vi "Run_2_of_6_Tests.vi"() -> ()   [LabVIEW 2019]
uses:
  <vilib>/Rock Robotics/WPI/ThirdParty/JAS_Junk/TrajLib/Trajectory_Library.lvlib
panel:
  out "Meca Drive \nOdometry":bool
  out "Meca Drive \nKinematics":bool
  out "String":string
  out "Flywheel Simulation":bool
  out "Matrix":bool
  out "PID":bool
  out "Math Utils":bool
  out "Linear Filter":bool
  out "Linear System Loop":bool
  out "All Tests Finished":bool
  out "Holonomic Drive Ctrl":bool
  out "Linear Plant Inv FF":bool
  out "Numerical Jacobian":bool
  out "Merwe Scaled Sigma Pts":bool
  out "Numerical Integration":bool
  out "Median Filter":bool
  out "Linear System ID":bool
  out "Kalman filter":bool
  out "PID Input / Output":bool
  out "Linear Quadradtic Regulator":bool
  # "FORMAL TRAJECTORY / CONTROL LIBRARY TEST PROCEDURE"
  # "FUNCTION NOT\nIMPLEMENTED"
  # "Extended Kalman Filter"
  # "FUNCTION NOT\nIMPLEMENTED"
  # "Meca Drive Pose Est"
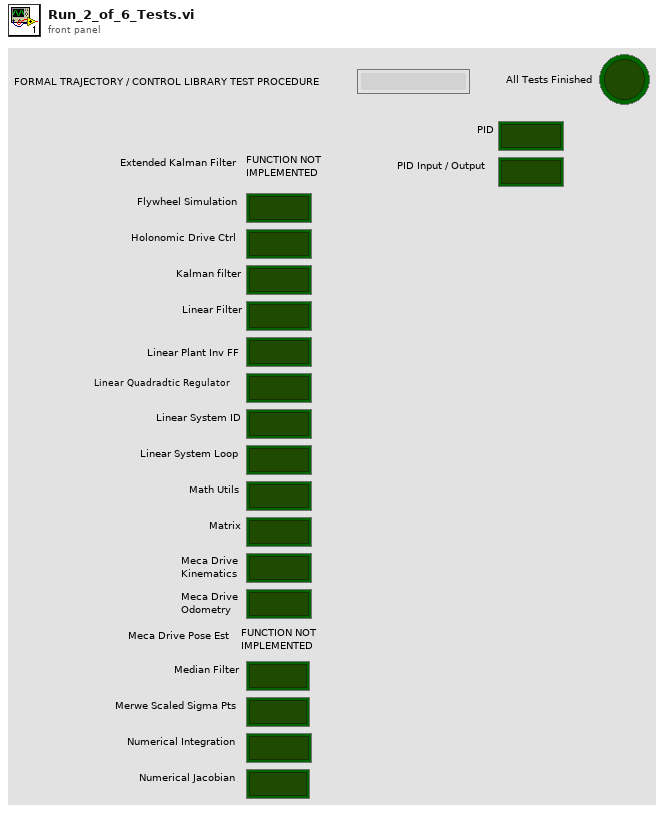
[diagram p1: front panel]
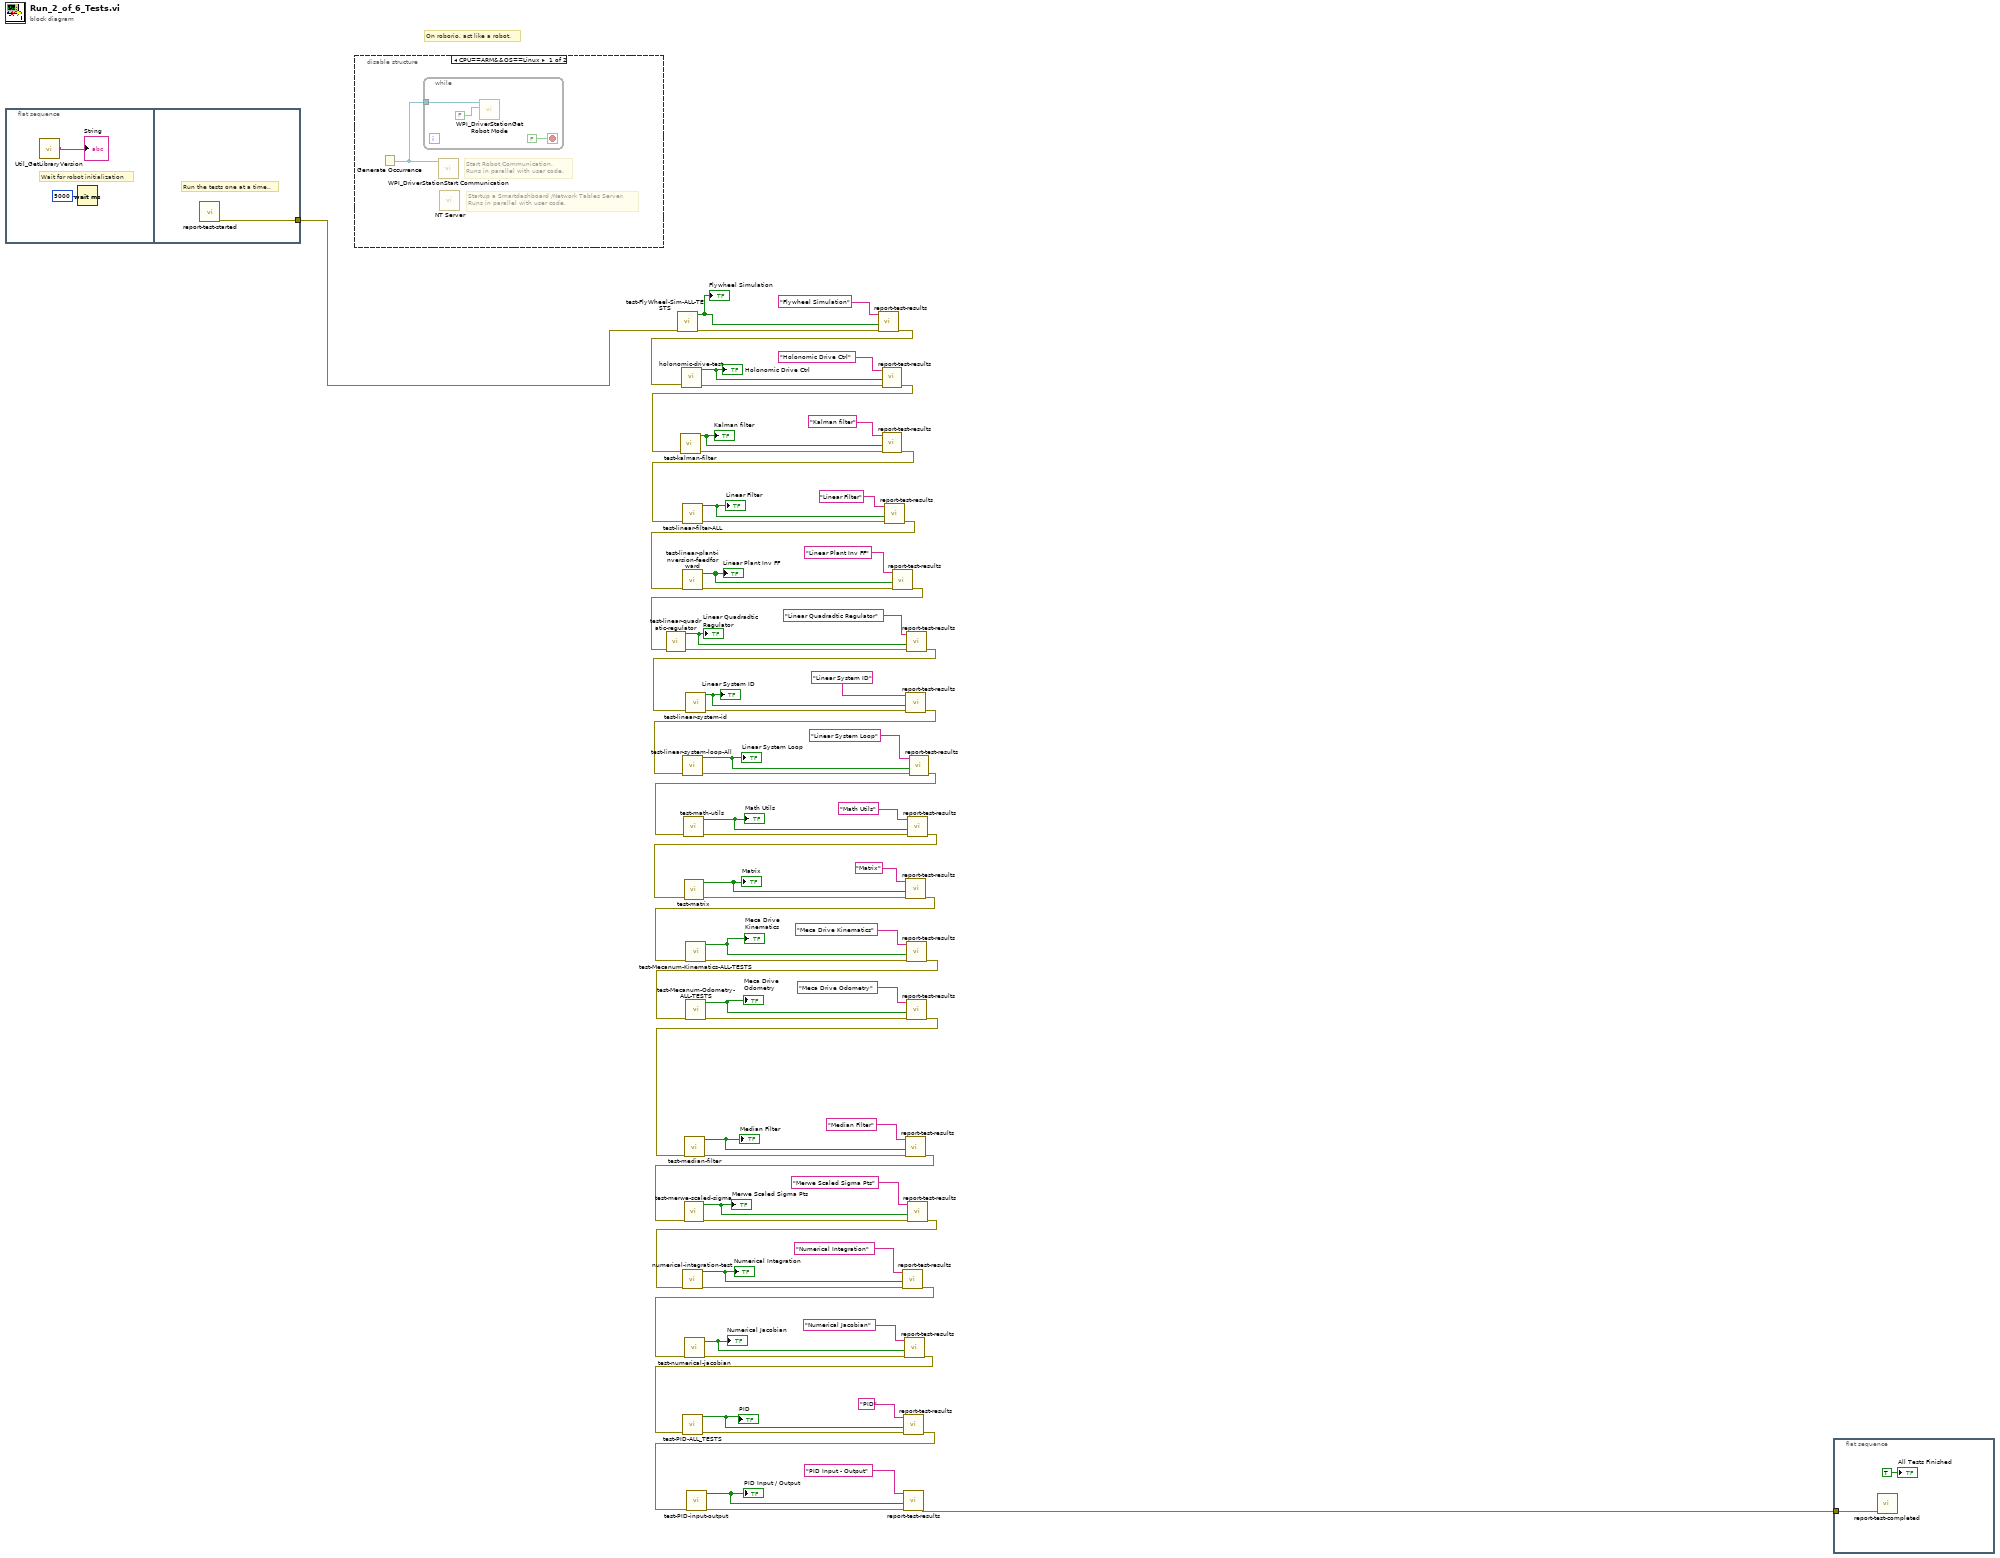
[diagram p0: block diagram]
diagram:
  # "On roborio, act like a robot."
  n1 = flat-sequence {
    tunnel: [w76] -> w12
    frame #0 {
      # "Wait for robot initialization"
      n2 = call <vilib>:"Util_GetLibraryVersion.vi"() -> ("TrajLibVersion"=→"String":string)  [unwired: 11 in]
      n3 = Wait (ms)(milliseconds to wait=u32 5000) -> ()  [unwired: 1 out]
    }
    frame #1 {
      # "Run the tests one at a time.."
      n4 = call "report-test-started.vi"() -> ("error out"=w76:errorcluster)  [unwired: 11 in]
    }
  }
  n5 = disable-structure shown="CPU==ARM&&OS==Linux" {
    frame condition #0 {
      # "Startup a Smartdashboard /Network Tables Server.\nRuns in parallel with user code."
      # "Start Robot Communication.\nRuns in parallel with user code."
      n6 = Generate Occurrence() -> (w77:refnum<k4>)
      n7 = while {
        tunnel: w77 -> [w80]
        stop <- FALSE stop-if-true
        n8 = call <vilib>:"WPI_DriverStationGet Robot Mode.vi"("Finish"=FALSE, "DS Occurrence"=w80) -> ()  [unwired: 10 out]
      }
      n9 = call <vilib>:"WPI_DriverStationStart Communication.vi"("occurrence"=w77) -> ()  [unwired: 2 in, 9 out]
      n10 = call <vilib>:"NT Server.vi"() -> ()  [unwired: 12 in]
    }
    frame condition #1 (active) {
    }
  }
  n11 = call "test-FlyWheel-Sim-ALL-TESTS.vi"("error in (no error)"=w12) -> ("error out"=w13:errorcluster, "All Passed"=w10:bool)  [unwired: 9 in]
  "Flywheel Simulation" <- w10
  n12 = call "report-test-results.vi"("error in (no error)"=w13, "TestPassed"=w10, "Test Name"="Flywheel Simulation") -> ("error out"=w11:errorcluster)  [unwired: 8 in]
  n13 = call "holonomic-drive-test.vi"("error in (no error)"=w11) -> ("error out"=w43:errorcluster, "ALL TESTS PASSED"=w71:bool)  [unwired: 9 in]
  "Holonomic Drive Ctrl" <- w71
  n14 = call "report-test-results.vi"("error in (no error)"=w43, "TestPassed"=w71, "Test Name"="Holonomic Drive Ctrl") -> ("error out"=w42:errorcluster)  [unwired: 8 in]
  n15 = call "test-kalman-filter.vi"("error in (no error)"=w42) -> ("error out"=w41:errorcluster, "ALL TESTS PASSED"=w70:bool)  [unwired: 9 in]
  "Kalman filter" <- w70
  n16 = call "report-test-results.vi"("error in (no error)"=w41, "TestPassed"=w70, "Test Name"="Kalman filter") -> ("error out"=w40:errorcluster)  [unwired: 8 in]
  n17 = call "test-linear-filter-ALL.vi"("error in (no error)"=w40) -> ("error out"=w38:errorcluster, "ALL TESTS GOOD"=w61:bool)  [unwired: 9 in]
  "Linear Filter" <- w61
  n18 = call "report-test-results.vi"("error in (no error)"=w38, "TestPassed"=w61, "Test Name"="Linear Filter") -> ("error out"=w37:errorcluster)  [unwired: 8 in]
  n19 = call "test-linear-plant-inversion-feedforward.vi"("error in (no error)"=w37) -> ("error out"=w36:errorcluster, "All Tests Passed"=w60:bool)  [unwired: 9 in]
  "Linear Plant Inv FF" <- w60
  n20 = call "report-test-results.vi"("error in (no error)"=w36, "TestPassed"=w60, "Test Name"="Linear Plant Inv FF") -> ("error out"=w35:errorcluster)  [unwired: 8 in]
  n21 = call "test-linear-quadratic-regulator.vi"("error in (no error)"=w35) -> ("error out"=w34:errorcluster, "ALL TESTS GOOD"=w59:bool)  [unwired: 9 in]
  "Linear Quadradtic Regulator" <- w59
  n22 = call "report-test-results.vi"("error in (no error)"=w34, "TestPassed"=w59, "Test Name"="Linear Quadradtic Regulator") -> ("error out"=w33:errorcluster)  [unwired: 8 in]
  n23 = call "test-linear-system-id.vi"("error in (no error)"=w33) -> ("error out"=w32:errorcluster, "All tests passed"=w58:bool)  [unwired: 9 in]
  "Linear System ID" <- w58
  n24 = call "report-test-results.vi"("error in (no error)"=w32, "TestPassed"=w58, "Test Name"="Linear System ID") -> ("error out"=w24:errorcluster)  [unwired: 8 in]
  n25 = call "test-linear-system-loop-All.vi"("error in (no error)"=w24) -> ("error out"=w25:errorcluster, "ALL TEsts Passed"=w57:bool)  [unwired: 9 in]
  "Linear System Loop" <- w57
  n26 = call "report-test-results.vi"("error in (no error)"=w25, "TestPassed"=w57, "Test Name"="Linear System Loop") -> ("error out"=w23:errorcluster)  [unwired: 8 in]
  n27 = call "test-math-utils.vi"("error in (no error)"=w23) -> ("error out"=w22:errorcluster, "ALL TESTS PASSED"=w56:bool)  [unwired: 9 in]
  "Math Utils" <- w56
  n28 = call "report-test-results.vi"("error in (no error)"=w22, "TestPassed"=w56, "Test Name"="Math Utils") -> ("error out"=w21:errorcluster)  [unwired: 8 in]
  n29 = call "test-matrix.vi"("error in (no error)"=w21) -> ("error out"=w26:errorcluster, "All Tests\nPassed"=w55:bool)  [unwired: 9 in]
  "Matrix" <- w55
  n30 = call "report-test-results.vi"("error in (no error)"=w26, "TestPassed"=w55, "Test Name"="Matrix") -> ("error out"=w6:errorcluster)  [unwired: 8 in]
  n31 = call "test-Mecanum-Kinematics-ALL-TESTS.vi"("error in (no error)"=w6) -> ("error out"=w8:errorcluster, "All Passed"=w7:bool)  [unwired: 9 in]
  "Meca Drive \nKinematics" <- w7
  n32 = call "report-test-results.vi"("error in (no error)"=w8, "TestPassed"=w7, "Test Name"="Meca Drive Kinematics") -> ("error out"=w2:errorcluster)  [unwired: 8 in]
  n33 = call "test-Mecanum-Odometry-ALL-TESTS.vi"("error in (no error)"=w2) -> ("error out"=w4:errorcluster, "All Passed"=w3:bool)  [unwired: 9 in]
  "Meca Drive \nOdometry" <- w3
  n34 = call "report-test-results.vi"("error in (no error)"=w4, "TestPassed"=w3, "Test Name"="Meca Drive Odometry") -> ("error out"=w1:errorcluster)  [unwired: 8 in]
  n35 = call "test-median-filter.vi"("error in (no error)"=w1) -> ("error out"=w27:errorcluster, "ALL TESTS PASSED"=w54:bool)  [unwired: 9 in]
  "Median Filter" <- w54
  n36 = call "report-test-results.vi"("error in (no error)"=w27, "TestPassed"=w54, "Test Name"="Median Filter") -> ("error out"=w20:errorcluster)  [unwired: 8 in]
  n37 = call "test-merwe-scaled-sigma.vi"("error in (no error)"=w20) -> ("error out"=w28:errorcluster, "All Tests Passed"=w44:bool)  [unwired: 9 in]
  "Merwe Scaled Sigma Pts" <- w44
  n38 = call "report-test-results.vi"("error in (no error)"=w28, "TestPassed"=w44, "Test Name"="Merwe Scaled Sigma Pts") -> ("error out"=w19:errorcluster)  [unwired: 8 in]
  n39 = call "numerical-integration-test.vi"("error in (no error)"=w19) -> ("error out"=w29:errorcluster, "All passed"=w45:bool)  [unwired: 9 in]
  "Numerical Integration" <- w45
  n40 = call "report-test-results.vi"("error in (no error)"=w29, "TestPassed"=w45, "Test Name"="Numerical Integration") -> ("error out"=w18:errorcluster)  [unwired: 8 in]
  n41 = call "test-numerical-jacobian.vi"("error in (no error)"=w18) -> ("error out"=w30:errorcluster, "ALL Tests Passed"=w46:bool)  [unwired: 9 in]
  "Numerical Jacobian" <- w46
  n42 = call "report-test-results.vi"("error in (no error)"=w30, "TestPassed"=w46, "Test Name"="Numerical Jacobian") -> ("error out"=w17:errorcluster)  [unwired: 8 in]
  n43 = call "test-PID-ALL_TESTS.vi"("error in (no error)"=w17) -> ("error out"=w31:errorcluster, "All Passed"=w47:bool)  [unwired: 9 in]
  "PID" <- w47
  n44 = call "report-test-results.vi"("error in (no error)"=w31, "TestPassed"=w47, "Test Name"="PID") -> ("error out"=w16:errorcluster)  [unwired: 8 in]
  n45 = call "test-PID-input-output.vi"("error in (no error)"=w16) -> ("error out"=w39:errorcluster, "All Passed"=w48:bool)  [unwired: 9 in]
  "PID Input / Output" <- w48
  n46 = call "report-test-results.vi"("error in (no error)"=w39, "TestPassed"=w48, "Test Name"="PID Input - Output") -> ("error out"=w15:errorcluster)  [unwired: 8 in]
  n47 = flat-sequence {
    tunnel: w15 -> [w81]
    frame #0 {
      n48 = call "report-test-completed.vi"("error in (no error)"=w81) -> ()  [unwired: 10 in, 1 out]
      "All Tests Finished" <- TRUE ("All Tests Finished")
    }
  }
